vi "SMSMagnet.SetValue.vi"(0 "i ref in":refnum<vi>, 2 "SetValue":dbl, 5 "error in (no error)":errorcluster) -> (14 "i ref out":refnum<vi>, 19 "error out":errorcluster)   [LabVIEW 2014, in "SMSMagnet.lvlib"]
doc: "This method serves to periodically do things like reading values from the HW. Methods that should be executed periodically should be called from THIS methode. Add code here."
uses:
  SMSMagnet.lvlib
  CS_Core/CSSystem/CoreDefs/CoreDefs.error_type.ctl
  CSlibraries-extern/DimLVEvent/LVDimInterface/LVDimInterface.lvlib
  CS_Core/CSSystem/CoreLib/CoreLib.lvlib
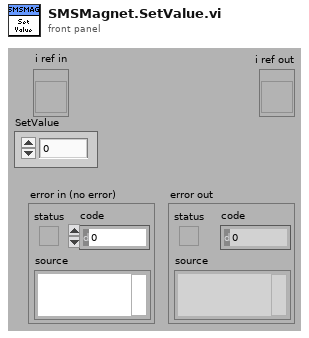
[diagram p1: front panel]
types:
  T1 = typedef "CoreDefs.error_type.ctl" = enum16{"no error", "can't load process", "can't unload process", "process does not exist", "can't install process", "can't remove process", "unknown function", "time out", "can't execute function", "duplicate queue name", "super not found", "caller queue invalid", "can't ping process", "unknown error", "VISA Error", "VISA timeout", "GPIB timeout", "GPIB error", "communication error", "data type mismatch", "can't read data from OPC server", "can't write data to OPC server", "OET error", "function not implemented", "process already exists", "invalid Shared Variable name", "error writing Shared Variable", "error reading Shared Variable", "invalid client name", "corrupt database", "unknown class", "call not authorized", "parameter out of range", "OET timeout: can't get data to modify", "invalid queue name", "requested operation incompatible with current state", "event undefined", "event disabled", "state undefined", "caller is not a friend", "EventBuilder: bad eventID", "EventBuilder: no DAQ devices", "a thread must not stop itself", "UNUSED ELEMENT4", "DiscArchiver: eventData incomplete", "DiscArchiver: eventData does not belong to run", "DiscArchiver: can't open file", "DiscArchiver: can't write to file", "DiscArchiver: available disc space low", "can't acquire semaphore", "error reading data from database", "notifier object is not existing", "can't register process", "can't unregister process", "illegal event type", "object disabled", "object already exists", "can't change state", "Instrument not found", "no connection to remote node", "invalid reference", "N/A", "UNUSED ELEMENT 1", "element not found", "illegal TCP/IP connection detected", "object does not exist", "invalid access ID", "unknown CS system", "invalid privilige", "unsupported data type", "unsupported server type", "IO server already exists", "Shared Variable already exists"}
  T2 = typedef "SMSMagnet.lvlib/SMSMagnet.i attribute.ctl" = cluster{"ActValueID":i32, "NomValueID":i32, "VISA resource name":refnum<visa-resource-name>, "ActValue":dbl, "VISAsem":T3}
  T3 = typedef "Semaphore RefNum" = refnum<k1>
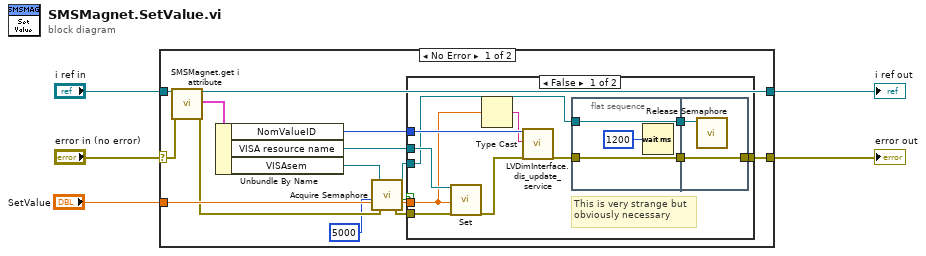
[diagram p0: block diagram]
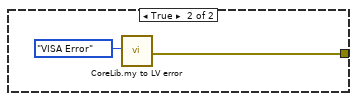
[diagram p2: hidden frame]
diagram:
  n1 = case shown="No Error" "error in (no error)" {
    selector: "error in (no error)" -> [w17 w38]
    tunnel: [w14 w38] -> w4
    tunnel: "i ref in" -> [w19 w39]
    tunnel: [w18 w39] -> w2
    tunnel: "SetValue" -> [w12 _]
    frame No Error {
      n2 = call "SMSMagnet.get i attribute.vi"("i ref in"=w19, "error in (no error)"=w17) -> ("i ref out"=w18:refnum<vi>, "i attribute"=w16:T2, "error out"=w10:errorcluster)  [unwired: 15 in]
      n3 = Unbundle By Name(w16) -> ("NomValueID"=w15:i32, "VISA resource name"=w13:refnum<visa-resource-name>, "VISAsem"=w11:T3)
      n4 = call <vilib>:"Acquire Semaphore.vi"("error in (no error)"=w10, "ms timeout (-1)"=5000, "semaphore"=w11) -> ("error out"=w9:errorcluster, "timed out"=w8:bool, "semaphore out"=w6:T3)  [unwired: 2 in]
      n5 = case shown="False" w8 {
        tunnel: w15 -> [w30 _]
        tunnel: [w23 w36] -> w14
        tunnel: w13 -> [w28 _]
        tunnel: w12 -> [w26 _]
        tunnel: w9 -> [w25 _]
        tunnel: w6 -> [w24 _]
        frame False {
          # "This is very strange but\nobviously necessary"
          n6 = call "Set.vi"("VISA resource name"=w28, "SetValue"=w26, "error in (no error)"=w25) -> ("error out"=w27:errorcluster)  [unwired: 15 in, 1 out]
          n7 = Type Cast(x=w26) -> (*(type *) &x=w29:string)  [unwired: 1 in]
          n8 = call "LVDimInterface.dis_update_service.vi"("my_serviceID"=w30, "data"=w29, "error in (no error)"=w27) -> ("error out"=w22:errorcluster)  [unwired: 14 in, 2 out]
          n9 = flat-sequence {
            tunnel: w22 -> [w32]
            tunnel: w24 -> [w33]
            tunnel: [w33] -> w21
            tunnel: [w32] -> w20
            tunnel: [w34] -> w23
            tunnel: w21 -> [w35]
            tunnel: w20 -> [w34]
            frame #0 {
              n10 = Wait (ms)(milliseconds to wait=u32 1200) -> ()  [unwired: 1 out]
            }
            frame #1 {
              n11 = call <vilib>:"Release Semaphore.vi"("semaphore"=w35) -> ()  [unwired: 5 in, 2 out]
            }
          }
        }
        frame True {
          n12 = call "CoreLib.my to LV error.vi"("ErrorTypes"=CoreDefs.error_type."VISA Error") -> ("myErrorCluster"=w36:errorcluster)  [unwired: 17 in, 1 out]
        }
      }
    }
    frame Error {
    }
  }
  "error out" <- w4
  "i ref out" <- w2
